vi "5 arduino lm35.vi"() -> ()   [LabVIEW 2015]
uses:
  <vilib>/LabVIEW Interface for Arduino/Type Defs/Analog Pin.ctl
  <vilib>/LabVIEW Interface for Arduino/Type Defs/Board Type.ctl
  <vilib>/LabVIEW Interface for Arduino/Type Defs/Connection Type.ctl
  <vilib>/LabVIEW Interface for Arduino/LabVIEW Interface for Arduino.lvlib
panel:
  out "Gauge":dbl(knob) scale=0.0..50.0
  out "Thermometer":dbl(slide) scale=0.0..100.0
  in  "Stop":bool
  in  "Analog Pin":T1
  out "ROOM TEMP":dbl
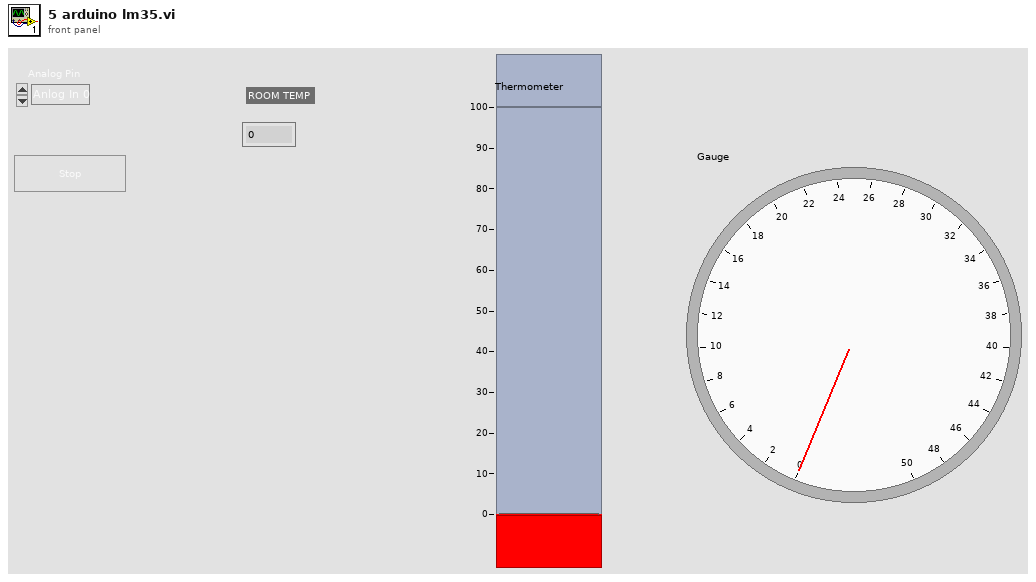
[diagram p1: front panel]
types:
  T1 = typedef "LabVIEW Interface for Arduino.lvlib/Analog Pin.ctl" = enum8{"Anlog In 0", "Anlog In 1", "Anlog In 2", "Anlog In 3", "Anlog In 4", "Anlog In 5"}
  T2 = typedef "LabVIEW Interface for Arduino.lvlib/Connection Type.ctl" = enum8{"USB / Serial", "XBEE", "BlueSmirf (Bluetooth)"}
  T3 = typedef "LabVIEW Interface for Arduino.lvlib/Board Type.ctl" = enum16{"Uno", "Dimuelanove w/Atmega 328", "Mega 2560"}
  T4 = typedef "LabVIEW Interface for Arduino.lvlib/Arduino Resource.ctl" = cluster{"VISA resource":refnum<visa-resource-name>, "Board Type":T3, "Connection Type":enum8{"USB / Serial"}, "Bytes Per Packet (15)":u8}
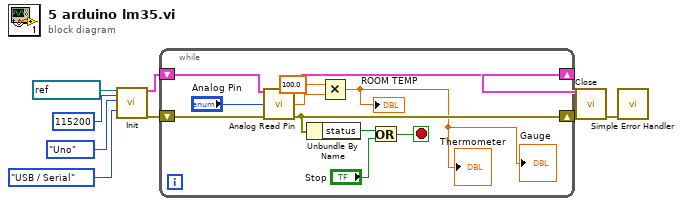
[diagram p0: block diagram]
diagram:
  n1 = call <vilib>:"Init.vi"("VISA resource"=refnum<visa-resource-name> "COM19", "Baud Rate (115200)"=u32 115200, "Board Type (Uno)"=Board_Type."Uno", "Connection Type (USB/Serial)"=Connection_Type."USB / Serial") -> ("Arduino Resource"=w9:T4, "error out"=w6:errorcluster)  [unwired: 14 in]
  n2 = while {
    shift-right: [w20] -> w8
    shift-left: w9 -> [w16]
    shift-right: [w19] -> w7
    shift-left: w6 -> [w15]
    stop <- w13 stop-if-true
    n3 = call <vilib>:"Analog Read Pin.vi"("Arduino Resource"=w16, "Analog Input Pin (0)"="Analog Pin", "error in"=w15) -> ("Arduino Resource"=w20:T4, "Voltage"=w12:dbl, "error out"=w19:errorcluster)  [unwired: 10 in]
    n4 = Unbundle By Name(w19) -> ("status"=w18:bool)
    n5 = Multiply(x=100.0, y=w12) -> (x*y=→"ROOM TEMP" →"Thermometer" →"Gauge":dbl)
    n6 = Or(x=w18, y="Stop") -> (x .or. y?=w13:bool)
  }
  n7 = call <vilib>:"Close.vi"("Arduino Resource"=w8, "error in"=w7) -> ("error out"=w5:errorcluster)  [unwired: 13 in]
  n8 = call <vilib>:"Simple Error Handler.vi"("error in (no error)"=w5) -> ()  [unwired: 4 in, 5 out]
